vi "Localization Mockup.vi"() -> ()   [LabVIEW 2015, in "Localization Mockup.lvlib"]
uses:
  Localization Mockup.lvlib
  PathfindingSettings.ctl
  MovementSettings.ctl
  PathCostWeights.ctl
  IntermediatePositionGrids.ctl
  Move.ctl
  <vilib>/Utility/miscctls.llb/LVBoundsTypeDef.ctl
  <vilib>/Utility/inputDevices.llb/mouseAcquire.vi
  Navigation2017-SubVIs.lvlib
  Navigation2017-util.lvlib
  Navigation2017.lvlib
panel:
  out "Heartbeat":bool=TRUE
  out "Move":T1={"Did Reach Dest"=FALSE, "Did Collide"=FALSE, "Sum of Angle Changes (rad)"=0.0, "Move Length (m)"=0.0, "Closeness Sum"=0.0, "Positions Along Move"=[{"x"=0.9948666606172851, "y"=1.2473033614636722, "angle"=1.6518517499971999}, {"x"=1.001713061664076, "y"=1.44718614409566, "angle"=1.536557632350141}, {"x"=1.031508296522137, "y"=1.644954301238697, "angle"=1.4212635147030823}, {"x"=1.0838567436054756, "y"=1.8379818642652317, "angle"=1.3059693970560236}, {"x"=1.158063319429836, "y"=2.0237058102291905, "angle"=1.1906752794089648}, {"x"=1.2531427079418764, "y"=2.199660093724013, "angle"=1.075381161761906}, {"x"=1.3678324435608575, "y"=2.363508391071432, "angle"=0.9600870441148471}, {"x"=1.5006096742160095, "y"=2.5130751220631486, "angle"=0.8447929264677883}, {"x"=1.6497113817997135, "y"=2.6463743373482496, "angle"=0.7294988088207294}, {"x"=1.8131577915490082, "y"=2.7616360878991832, "angle"=0.6142046911736705}, {"x"=1.988778659525295, "y"=2.8573299264221292, "angle"=0.49891057352661167}, {"x"=2.1742420891466807, "y"=2.9321852286596677, "angle"=0.38361645587955284}, {"x"=2.367085494146603, "y"=2.9852080647591808, "angle"=0.268322338232494}, {"x"=2.564748296832094, "y"=3.0156943966887, "angle"=0.1530282205854352}, {"x"=2.7646059274737063, "y"=3.0232394264647042, "angle"=0.037734102938376354}, {"x"=2.9640046733826884, "y"=3.007742971065964, "angle"=-0.07756001470868248}, {"x"=3.1602969149488147, "y"=2.969410792665233, "angle"=-0.19285413235574134}, {"x"=3.350876280774229, "y"=2.90875186651596, "angle"=-0.30814825000280016}, {"x"=3.5332122551128893, "y"=2.8265716227710582, "angle"=-0.423442367649859}, {"x"=3.704883778097503, "y"=2.7239612519689644, "angle"=-0.5387364852969179}, {"x"=3.863611392609625, "y"=2.6022832161889142, "angle"=-0.6540306029439767}, {"x"=4.007287510946279, "y"=2.4631531582585313, "angle"=-0.7693247205910356}, {"x"=4.134004399401844, "y"=2.3084184492235513, "angle"=-0.8846188382380945}, {"x"=4.134004399401844, "y"=2.3084184492235513, "angle"=5.398566468941492}], "Moved Fwd"=TRUE}
  in  "Specify End Angle":bool
  in  "Pathfinding Settings":T2={"Movement Settings"={"Arrival Tolerance (m)"=0.01, "Closeness Threshold (m)"=0.5, "Pit Obstacle Radius (m)"=0.5, "Pit Locations"=[]}, "Dead Zone"=0.75, "Max Moves"=3.0, "Move Segment Length (m)"=0.2, "Path Cost Weights"={"Length Weight"=1.0, "Angle Weight"=0.0, "Angle Error Weight"=1000.0, "Angle Error Threshold"=0.314, "Per Move Penalty"=0.05, "Closeness Weight"=100.0, "Too Short Penalty"=100.0, "Too Short Threshold"=1.5}, "Desperation - Reduction Per Attempt (Ratio)"=0.9, "Desperation - Max Attempts"=1, "Log All Move Points"=FALSE, "Intermediate Position Grids"=[{"x1"=0.0, "x2"=1.75, "resolution"=0.15}, {"x1"=1.75, "x2"=7.38, "resolution"=0.4}]}
  in  "Full Pathfinding":bool=TRUE
  in  "Choose Background":u16
  out "Numeric 4":dbl=2.9395922017001697
  out "Numeric 3":dbl=2.276578752456705
  out "Numeric 2":dbl=2.7971305825546784
  out "Numeric":dbl=2.0893893844143916
  in  "Speed":dbl(slide) scale=0.0..1.0
  in  "Turning Radius":dbl(slide)=1.7346938775510203 scale=1.0..10.0
  out "Dest Y":dbl
  out "Dest X":dbl
  in  "ACTUALLY SEND VALUES TO ROBOT":bool
  in  "Send Robot STOP, end program":bool
  out "Left Side PWM":dbl=0.5
  out "Right Side PWM":dbl=0.5
  out "Bot Y (m)":dbl=1.04796
  out "Bot X (m)":dbl=1.01106
  out "Mouse Button Down":dbl
  out "Mouse Down":bool
  out "Bot Angle":dbl=1.7671458676442586
  out "Mouse Y (m)":dbl
  out "Mouse X (m)":dbl=0.08856
  out "Arena Control - DO NOT MOVE":picture
  # "\"missing\" side of robot faces forward (i.e. camera-side, boxes in back)"
  # "CONTROLS:\nClick + Drag to Move Robot\nMouse Wheel to Spin Robot\nRight Click to Place Yellow Destination Puck"
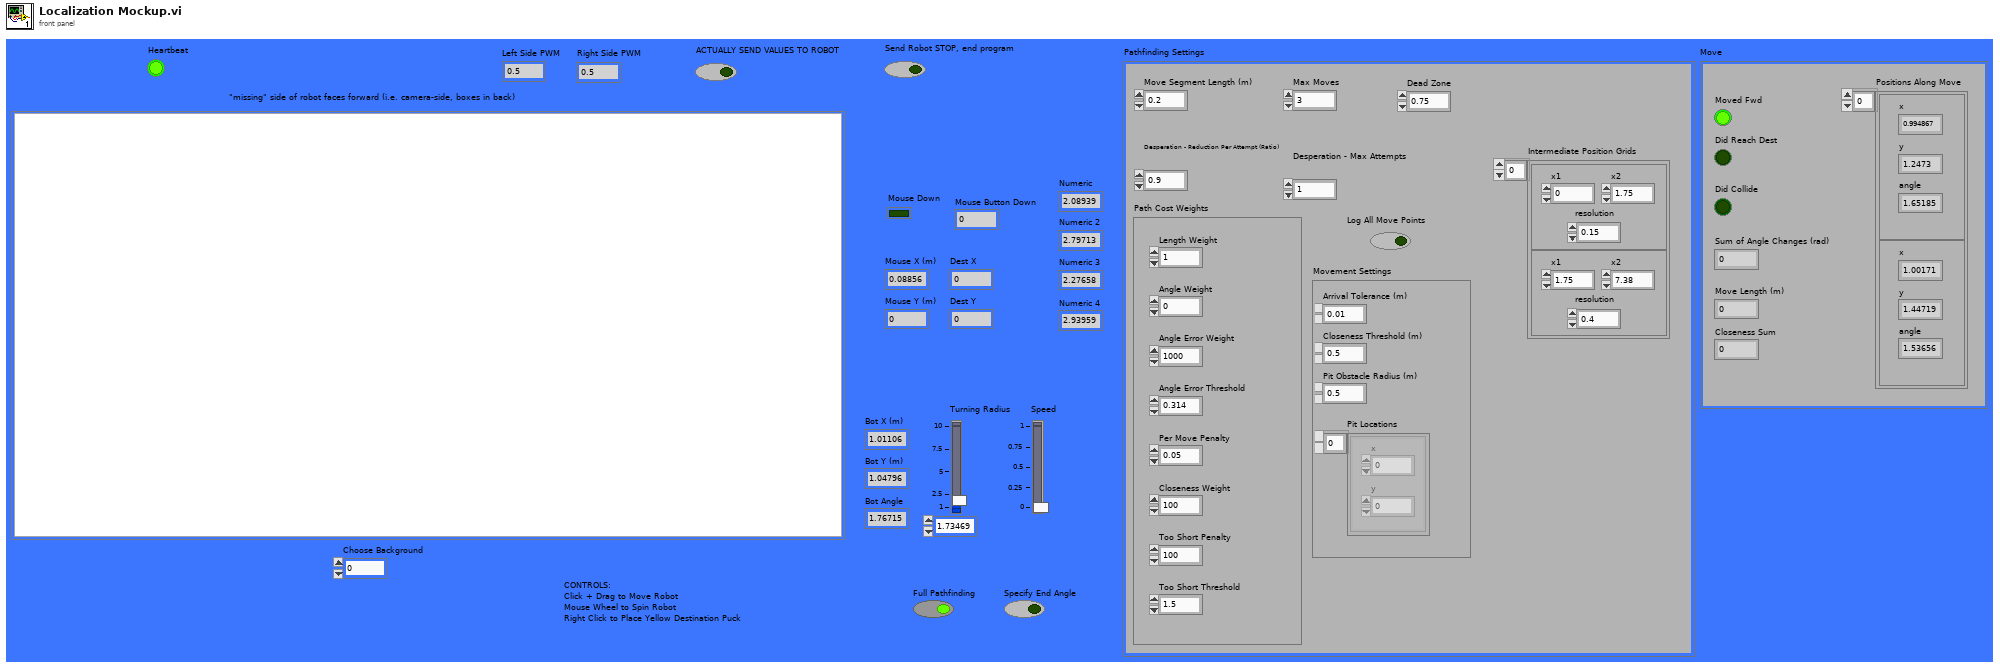
[diagram p1: front panel]
types:
  T1 = typedef "Navigation2017.lvlib/Move.ctl" = cluster{"Did Reach Dest":bool, "Did Collide":bool, "Sum of Angle Changes (rad)":dbl, "Move Length (m)":dbl, "Closeness Sum":dbl, "Positions Along Move":cluster{"x":dbl, "y":dbl, "angle":dbl}[], "Moved Fwd":bool}
  T2 = typedef "Navigation2017.lvlib/PathfindingSettings.ctl" = cluster{"Movement Settings":T3, "Dead Zone":dbl, "Max Moves":dbl, "Move Segment Length (m)":dbl, "Path Cost Weights":T4, "Desperation - Reduction Per Attempt (Ratio)":dbl, "Desperation - Max Attempts":i16, "Log All Move Points":bool, "Intermediate Position Grids":T5}
  T3 = typedef "Navigation2017.lvlib/MovementSettings.ctl" = cluster{"Arrival Tolerance (m)":dbl, "Closeness Threshold (m)":dbl, "Pit Obstacle Radius (m)":dbl, "Pit Locations":cluster{"x":dbl, "y":dbl}[]}
  T4 = typedef "Navigation2017.lvlib/PathCostWeights.ctl" = cluster{"Length Weight":dbl, "Angle Weight":dbl, "Angle Error Weight":dbl, "Angle Error Threshold":dbl, "Per Move Penalty":dbl, "Closeness Weight":dbl, "Too Short Penalty":dbl, "Too Short Threshold":dbl}
  T5 = typedef "Navigation2017.lvlib/IntermediatePositionGrids.ctl" = cluster{"x1":dbl, "x2":dbl, "resolution":dbl}[]
  T6 = typedef "LVBoundsTypeDef.ctl" = cluster{"Width":u32, "Height":u32}
  T7 = typedef "imagedata.ctl" = cluster{"image type":i32, "image depth":i32, "image":u8[], "mask":u8[], "colors":u32[], "Rectangle":cluster{"left":i16, "top":i16, "right":i16, "bottom":i16}}
  T8 = cluster{"Width":u16, "Style":enum32{"Solid", "Dash", "Dot", "DashDot", "DashDotDot"}}
  T9 = cluster{"Arrival Tolerance (m)":dbl, "Closeness Threshold (m)":dbl, "Pit Obstacle Radius (m)":dbl, "Pit Locations":cluster{"x":dbl, "y":dbl}[]}
  T10 = cluster{"Horizontal":i32, "Vertical":i32, "Scrolling":i32}
  T11 = typedef "LVRectTypeDef.ctl" = cluster{"Left":i16, "Top":i16, "Right":i16, "Bottom":i16}
  T12 = typedef "LVPointTypeDef.ctl" = cluster{"Horizontal":i16, "Vertical":i16}
  T13 = typedef "LVPositionTypeDef.ctl" = cluster{"Left":i32, "Top":i32}
  T14 = cluster{"Mouse X (m)":dbl, "Mouse Y (m)":dbl, dbl}
  T15 = typedef "Navigation2017.lvlib/Path.ctl" = cluster{"Dest Angle Error":dbl, "Dest Angle Considered":bool, "Moves":T1[]}
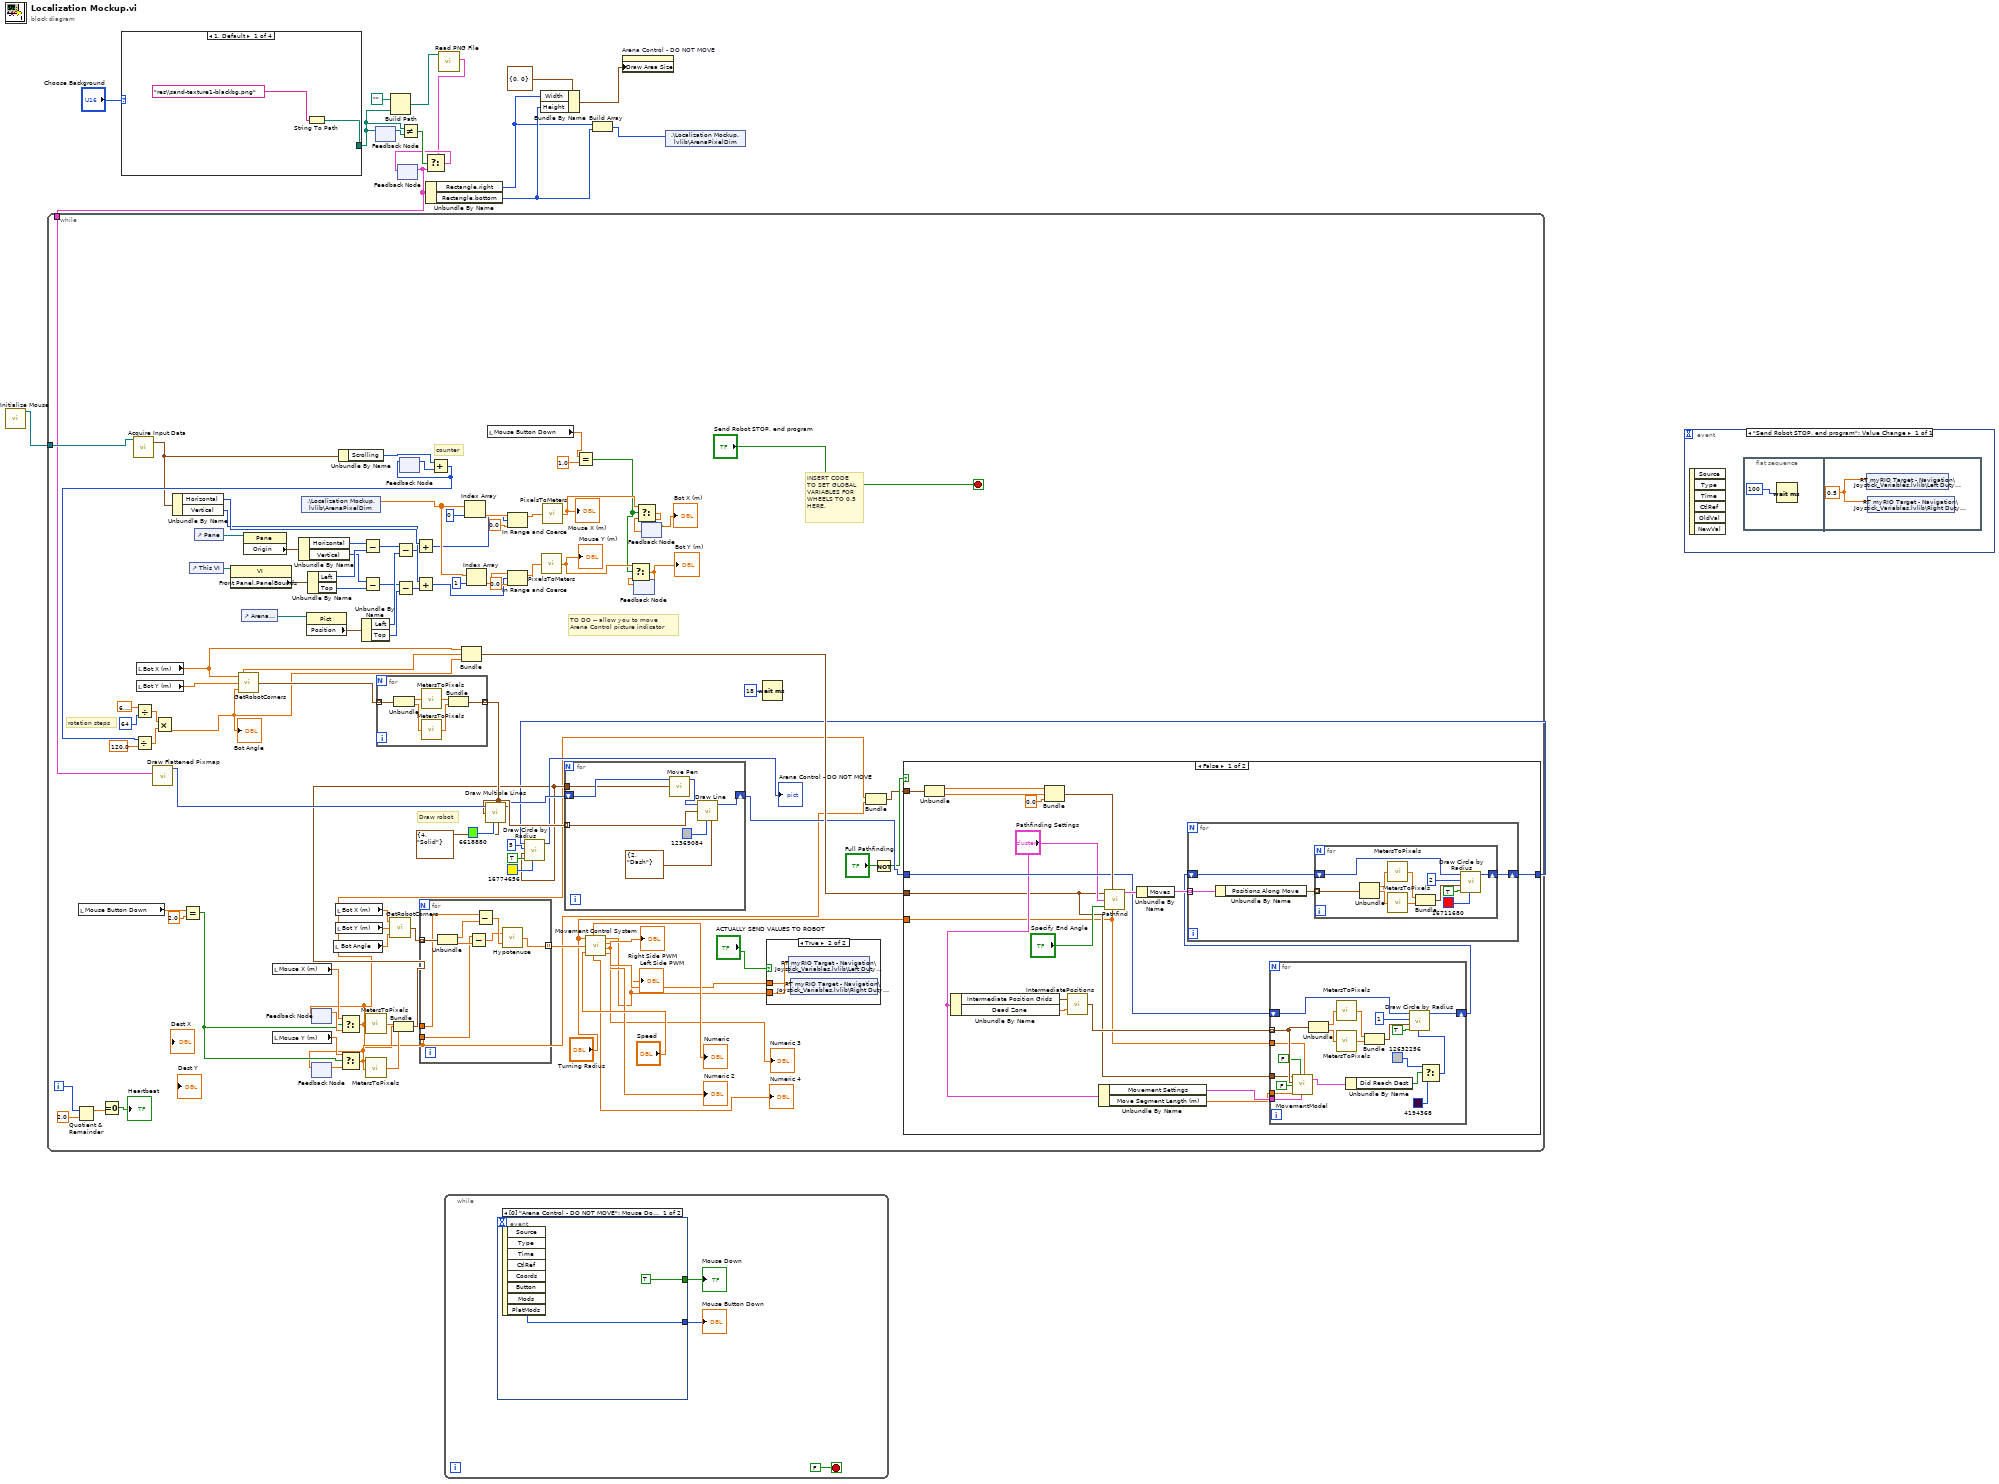
[diagram p0: block diagram]
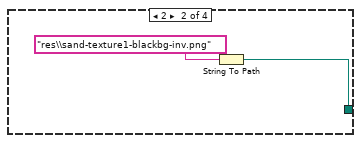
[diagram p2: hidden frame]
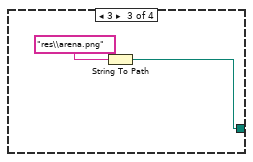
[diagram p3: hidden frame]
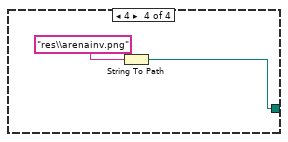
[diagram p4: hidden frame]
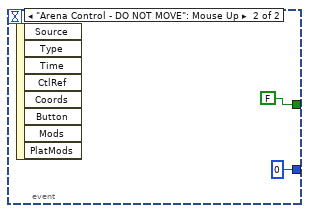
[diagram p5: hidden frame]
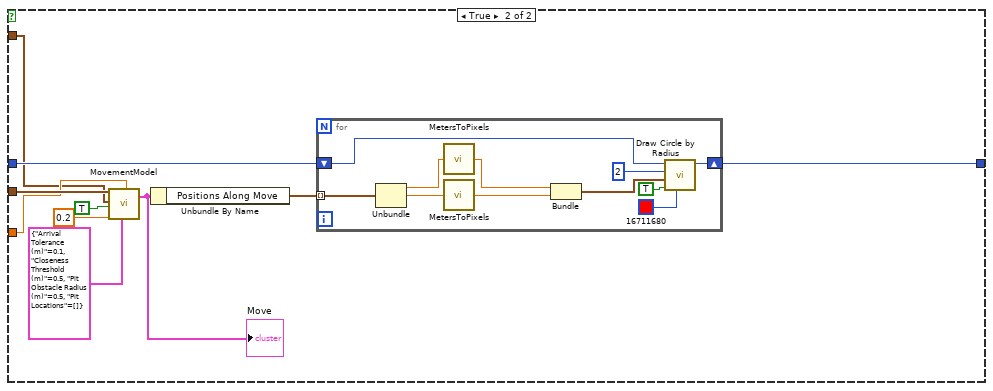
[diagram p6: hidden frame]
diagram:
  n1 = call <vilib>:"Initialize Mouse.vi"() -> ("device ID"=w15:refnum<k1>)  [unwired: 10 in, 1 out]
  n2 = case shown="1, Default" "Choose Background" {
    tunnel: [w16 w18 w20 w22] -> w10
    frame 1, Default {
      n3 = String To Path(string="res\\sand-texture1-blackbg.png" ("name or relative path")) -> (path=w16:path)
    }
    frame 2 {
      n4 = String To Path(string="res\\sand-texture1-blackbg-inv.png" ("name or relative path")) -> (path=w18:path)
    }
    frame 3 {
      n5 = String To Path(string="res\\arena.png" ("name or relative path")) -> (path=w20:path)
    }
    frame 4 {
      n6 = String To Path(string="res\\arenainv.png" ("name or relative path")) -> (path=w22:path)
    }
  }
  n7 = feedback #1() -> (w11:path)  [unwired: 1 in]
  n8 = feedback-in #1(w10) -> ()
  n9 = Build Path(base path=path "", name or relative path=w10) -> (appended path=w2:path)
  n10 = feedback #2() -> (w1:T7)  [unwired: 1 in]
  n11 = while {
    tunnel: w15 -> [w123]
    tunnel: w1 -> [w42]
    i -> [w34]
    stop <- "Send Robot STOP, end program" stop-if-true
    # "TO DO -- allow you to move\nArena Control picture indicator"
    # "INSERT CODE\nTO SET GLOBAL\nVARIABLES FOR\nWHEELS TO 0.5\nHERE."
    # "Draw robot"
    # "rotation steps"
    # "counter"
    n12 = Quotient & Remainder(x=w34, y=2.0) -> (x-y*floor(x/y)=w33:dbl)  [unwired: 1 out]
    n13 = local read "Mouse Button Down"() -> (w81:dbl)
    n14 = Equal To 0?(x=w33) -> (x = 0?=→"Heartbeat":bool)
    n15 = call-poly <vilib>:"Acquire Input Data.vi"("device ID"=w123) -> ("axis info"=w25:T10)  [unwired: 15 in, 3 out]
    n16 = Divide(x=6.283185307179586, y=64) -> (x/y=w95:dbl)
    n17 = local read "Bot X (m)"() -> (w49:dbl)
    n18 = local read "Bot Y (m)"() -> (w48:dbl)
    n19 = call <vilib>:"Draw Flattened Pixmap.vi"("image data"=w42) -> ("new picture"=w104:picture)  [unwired: 8 in]
    n20 = Unbundle By Name(w25) -> ("Horizontal"=w114:i32, "Vertical"=w113:i32)
    n21 = Equal?(x=w81, y=2.0) -> (x = y?=w71:bool)
    n22 = control-ref of="This VI"() -> (w61:refnum<vi>)
    n23 = control-ref of="Pane"() -> (w121:refnum<vi>)
    n24 = property class="VI"(reference=w61) -> ("Front Panel.PanelBounds"=w119:T11)  [unwired: 1 in, 2 out]
    n25 = control-ref of="Arena Control"() -> (w60:refnum<vi>)
    n26 = property class="Pane"(reference=w121) -> ("Origin"=w120:T12)  [unwired: 1 in, 2 out]
    n27 = local read "Mouse X (m)"() -> (w72:dbl)
    n28 = local read "Mouse Y (m)"() -> (w73:dbl)
    n29 = Unbundle By Name(w120) -> ("Horizontal"=w118:i16, "Vertical"=w116:i16)
    n30 = shared-variable ".\\Localization Mockup.lvlib\\ArenaPixelDim"() -> (w108:dbl[])  [unwired: 1 in, 1 out]
    n31 = property class="Pict"(reference=w60) -> ("Position"=w59:T13)  [unwired: 1 in, 2 out]
    n32 = Unbundle By Name(w119) -> ("Left"=w117:i16, "Top"=w115:i16)
    n33 = feedback #3() -> (w80:dbl)  [unwired: 1 in]
    n34 = feedback #4() -> (w79:dbl)  [unwired: 1 in]
    n35 = local read "Bot Angle"() -> (w76:dbl)
    n36 = local read "Bot X (m)"() -> (w69:dbl)
    n37 = local read "Bot Y (m)"() -> (w70:dbl)
    n38 = Unbundle By Name(w25) -> ("Scrolling"=w24:i32)
    n39 = Select(t=w72, s=w71, f=w80) -> (s? t:f=w37:dbl)
    n40 = feedback-in #3(w37) -> ()
    n41 = Select(t=w73, s=w71, f=w79) -> (s? t:f=w38:dbl)
    n42 = feedback-in #4(w38) -> ()
    n43 = Unbundle By Name(w59) -> ("Left"=w29:i32, "Top"=w26:i32)
    n44 = Subtract(x=w118, y=w117) -> (x-y=w30:i16)
    n45 = Subtract(x=w116, y=w115) -> (x-y=w27:i16)
    n46 = call "MetersToPixels.vi"("Arena Meters"=w37) -> ("Arena Pixels"=w64:dbl)
    n47 = call "MetersToPixels.vi"("Arena Meters"=w38) -> ("Arena Pixels"=w65:dbl)
    n48 = call "GetRobotCorners.vi"("botAngle (rad)"=w76, "botY (m)"=w70, "botX (m)"=w69) -> ("Corner Points (m)"=w78:cluster{dbl, dbl}[])
    n49 = Bundle("Arena Pixels"=w64, "Arena Pixels"=w65) -> (w45:cluster{"Arena Pixels":dbl, "Arena Pixels":dbl})  [unwired: 1 in]
    n50 = Subtract(x=w30, y=w29) -> (x-y=w31:i32)
    n51 = Subtract(x=w27, y=w26) -> (x-y=w28:i32)
    n52 = feedback #5() -> (w122:i32)  [unwired: 1 in]
    n53 = Add(x=w114, y=w31) -> (x+y=w58:i32)
    n54 = Add(x=w113, y=w28) -> (x+y=w57:i32)
    n55 = for {
      tunnel: w78 -> [w209] mode=indexing
      tunnel: [w204] -> w77 mode=indexing
      tunnel: w37 -> [w203]
      tunnel: w38 -> [w202]
      n56 = Unbundle(w209) -> (w208:dbl, w205:dbl)
      n57 = Subtract(x=w202, y=w205) -> (x-y=w206:dbl)
      n58 = Subtract(x=w203, y=w208) -> (x-y=w207:dbl)
      n59 = call "Hypotenuse.vi"("y"=w207, "x"=w206) -> ("r"=w204:dbl)
    }
    n60 = Add(x=w24, y=w122) -> (x+y=w94:i32)
    n61 = Divide(x=w94, y=120.0) -> (x/y=w101:dbl)
    n62 = Multiply(x=w95, y=w101) -> (x*y=w47:dbl)
    "Bot Angle" <- w47
    n63 = call "GetRobotCorners.vi"("botAngle (rad)"=w47, "botY (m)"=w48, "botX (m)"=w49) -> ("Corner Points (m)"=w93:cluster{dbl, dbl}[])
    n64 = for {
      tunnel: [w222] -> w92 mode=indexing
      tunnel: w93 -> [w221] mode=indexing
      n65 = Unbundle(w221) -> (w220:dbl, w217:dbl)
      n66 = call "MetersToPixels.vi"("Arena Meters"=w220) -> ("Arena Pixels"=w219:dbl)
      n67 = call "MetersToPixels.vi"("Arena Meters"=w217) -> ("Arena Pixels"=w218:dbl)
      n68 = Bundle("Arena Pixels"=w219, "Arena Pixels"=w218) -> (w222:cluster{"Arena Pixels":dbl, "Arena Pixels":dbl})  [unwired: 1 in]
    }
    n69 = feedback-in #5(w94) -> ()
    n70 = Bundle("Bot X (m)"=w49, "Bot Y (m)"=w48, w47) -> (w46:cluster{"Bot X (m)":dbl, "Bot Y (m)":dbl, dbl})  [unwired: 1 in]
    n71 = Index Array(array=w108, index=0) -> (element=w110:dbl)
    n72 = Index Array(array=w108, index=1) -> (element=w106:dbl)
    n73 = call <vilib>:"Draw Multiple Lines.vi"("picture"=w104, "line endpoints"=w92, "color(black)"=u32 6618880, "pen"=T8 {"Width"=4, "Style"=enum."Solid"}) -> ("new picture"=w63:picture)  [unwired: 5 in]
    n74 = local read "Mouse Button Down"() -> (w90:dbl)
    n75 = In Range and Coerce(upper limit=w110, x=w58, lower limit=0.0) -> (coerced(x)=w100:dbl)  [unwired: 1 out]
    n76 = In Range and Coerce(upper limit=w106, x=w57, lower limit=0.0) -> (coerced(x)=w99:dbl)  [unwired: 1 out]
    n77 = call "PixelsToMeters.vi"("Arena Meters"=w99) -> ("Arena Pixels"=w85:dbl)
    "Mouse Y (m)" <- w85
    n78 = call "PixelsToMeters.vi"("Arena Meters"=w100) -> ("Arena Pixels"=w89:dbl)
    "Mouse X (m)" <- w89
    n79 = for {
      tunnel: w92 -> [w213] mode=indexing
      shift-right: [w214] -> w43
      shift-left: w63 -> [w215]
      tunnel: w45 -> [w210]
      n80 = call <vilib>:"Move Pen.vi"("new position"=w210, "picture"=w215) -> ("new picture"=w216:picture)  [unwired: 3 in]
      n81 = call <vilib>:"Draw Line.vi"("picture"=w216, "end point"=w213, "color(black)"=u32 12369084, "pen"=T8 {"Width"=2, "Style"=enum."Dash"}) -> ("new picture"=w214:picture)  [unwired: 5 in]
    }
    n82 = Equal?(x=w90, y=1.0) -> (x = y?=w84:bool)
    n83 = call "Movement Control System.vi"("Turning Radius"="Turning Radius", "Corner Distances"=w77, "Speed"="Speed") -> ("Corner Dist 1"=→"Numeric":dbl, "Corner Dist 4"=→"Numeric 4":dbl, "Left Side PWM"=w51:dbl, "Corner Dist 2"=→"Numeric 2":dbl, "Right Side PWM"=w54:dbl, "Corner Dist 3"=→"Numeric 3":dbl)
    "Right Side PWM" <- w54
    "Left Side PWM" <- w51
    n84 = feedback #6() -> (w88:dbl)  [unwired: 1 in]
    n85 = Select(t=w85, s=w84, f=w88) -> (s? t:f=w83:dbl)
    "Bot Y (m)" <- w83
    n86 = feedback-in #6(w83) -> ()
    n87 = feedback #7() -> (w86:dbl)  [unwired: 1 in]
    "Bot X (m)" <- w86
    n88 = Select(t=w89, s=w84, f=w86) -> (s? t:f=w87:dbl)
    n89 = feedback-in #7(w87) -> ()
    n90 = Wait (ms)(milliseconds to wait=u32 18) -> ()  [unwired: 1 out]
    n91 = case shown="True" "ACTUALLY SEND VALUES TO ROBOT" {
      tunnel: w51 -> [_ w201]
      tunnel: w54 -> [_ w200]
      frame False {
      }
      frame True {
        n92 = shared-variable "RT myRIO Target - Navigation\\Joystick_Variables.lvlib\\Left Duty Cycle"(w201) -> ()  [unwired: 1 in, 1 out]
        n93 = shared-variable "RT myRIO Target - Navigation\\Joystick_Variables.lvlib\\Right Duty Cycle"(w200) -> ()  [unwired: 1 in, 1 out]
      }
    }
    n94 = Bundle("Mouse X (m)"=w37, "Mouse Y (m)"=w38) -> (w36:cluster{"Mouse X (m)":dbl, "Mouse Y (m)":dbl})  [unwired: 1 in]
    n95 = Not(x="Full Pathfinding") -> (.not. x?=w39:bool)
    n96 = case shown="False" w39 {
      tunnel: w46 -> [w125 w188]
      tunnel: [w142 w187] -> w44
      tunnel: w43 -> [w132 w186]
      tunnel: "Turning Radius" -> [w124 w181]
      tunnel: w36 -> [w136 w180]
      frame False {
        n97 = Unbundle(w136) -> ("Mouse X (m)"=w137:dbl, "Mouse Y (m)"=w135:dbl)
        n98 = Unbundle By Name("Pathfinding Settings") -> ("Intermediate Position Grids"=w130:T5, "Dead Zone"=w129:dbl)
        n99 = Bundle("Mouse X (m)"=w137, "Mouse Y (m)"=w135, 0.0) -> (w138:T14)  [unwired: 1 in]
        n100 = call "IntermediatePositions.vi"("Dead Zone"=w129, "Position Grids"=w130) -> ("Positions"=w131:cluster{dbl, dbl}[])
        n101 = Unbundle By Name("Pathfinding Settings") -> ("Movement Settings"=w127:T3, "Move Segment Length (m)"=w126:dbl)
        n102 = call "Pathfind.vi"("Start Vector"=w125, "Destination"=w138, "Pathfinding Settings"="Pathfinding Settings", "Specified End Angle"="Specify End Angle", "Turn Radius (m)"=w124) -> ("Best Path"=w141:T15)  [unwired: 3 out]
        n103 = Unbundle By Name(w141) -> ("Moves"=w140:T1[])
        n104 = for {
          shift-right: [w163] -> w133
          shift-left: w132 -> [w162]
          tunnel: w131 -> [w146] mode=indexing
          tunnel: w127 -> [w149]
          tunnel: w126 -> [w148]
          tunnel: w125 -> [w145]
          tunnel: w124 -> [w143]
          n105 = call "MovementModel.vi"("Start Vector"=w145, "Destination"=w146, "Log All Points"=FALSE, "Segment Length (m)"=w148, "Do Force Direction"=FALSE, "Movement Settings"=w149, "Turn Radius (m)"=w143) -> ("Move"=w154:T1)  [unwired: 11 in, 1 out]
          n106 = Unbundle(w146) -> (w159:dbl, w158:dbl)
          n107 = call "MetersToPixels.vi"("Arena Meters"=w159) -> ("Arena Pixels"=w157:dbl)
          n108 = call "MetersToPixels.vi"("Arena Meters"=w158) -> ("Arena Pixels"=w156:dbl)
          n109 = Unbundle By Name(w154) -> ("Did Reach Dest"=w153:bool)
          n110 = Bundle("Arena Pixels"=w157, "Arena Pixels"=w156) -> (w155:cluster{"Arena Pixels":dbl, "Arena Pixels":dbl})  [unwired: 1 in]
          n111 = Select(t=u32 12632256 ("color(black)"), s=w153, f=u32 4194368 ("color(black)")) -> (s? t:f=w151:u32)
          n112 = call <vilib>:"Draw Circle by Radius.vi"("color(black)"=w151, "fill?(F)"=TRUE, "pixel center"=w155, "radius"=i16 1, "picture"=w162) -> ("new picture"=w163:picture)  [unwired: 6 in]
        }
        n113 = for {
          shift-right: [w167] -> w142
          shift-left: w133 -> [w166]
          tunnel: w140 -> [w165] mode=indexing
          n114 = Unbundle By Name(w165) -> ("Positions Along Move"=w164:cluster{"x":dbl, "y":dbl, "angle":dbl}[])
          n115 = for {
            shift-right: [w175] -> w167
            shift-left: w166 -> [w174]
            tunnel: w164 -> [w173] mode=indexing
            n116 = Unbundle(w173) -> ("x"=w172:dbl, "y"=w171:dbl)  [unwired: 1 out]
            n117 = call "MetersToPixels.vi"("Arena Meters"=w172) -> ("Arena Pixels"=w170:dbl)
            n118 = call "MetersToPixels.vi"("Arena Meters"=w171) -> ("Arena Pixels"=w169:dbl)
            n119 = Bundle("Arena Pixels"=w170, "Arena Pixels"=w169) -> (w168:cluster{"Arena Pixels":dbl, "Arena Pixels":dbl})  [unwired: 1 in]
            n120 = call <vilib>:"Draw Circle by Radius.vi"("color(black)"=u32 16711680, "fill?(F)"=TRUE, "pixel center"=w168, "radius"=i16 2, "picture"=w174) -> ("new picture"=w175:picture)  [unwired: 6 in]
          }
        }
      }
      frame True {
        n121 = call "MovementModel.vi"("Start Vector"=w188, "Destination"=w180, "Log All Points"=TRUE, "Segment Length (m)"=0.2, "Movement Settings"=T9 {"Arrival Tolerance (m)"=0.1, "Closeness Threshold (m)"=0.5, "Pit Obstacle Radius (m)"=0.5, "Pit Locations"=[]}, "Turn Radius (m)"=w181) -> ("Move"=w184:T1)  [unwired: 12 in, 1 out]
        "Move" <- w184
        n122 = Unbundle By Name(w184) -> ("Positions Along Move"=w185:cluster{"x":dbl, "y":dbl, "angle":dbl}[])
        n123 = for {
          shift-right: [w196] -> w187
          shift-left: w186 -> [w195]
          tunnel: w185 -> [w194] mode=indexing
          n124 = Unbundle(w194) -> ("x"=w193:dbl, "y"=w192:dbl)  [unwired: 1 out]
          n125 = call "MetersToPixels.vi"("Arena Meters"=w193) -> ("Arena Pixels"=w191:dbl)
          n126 = call "MetersToPixels.vi"("Arena Meters"=w192) -> ("Arena Pixels"=w190:dbl)
          n127 = Bundle("Arena Pixels"=w191, "Arena Pixels"=w190) -> (w189:cluster{"Arena Pixels":dbl, "Arena Pixels":dbl})  [unwired: 1 in]
          n128 = call <vilib>:"Draw Circle by Radius.vi"("color(black)"=u32 16711680, "fill?(F)"=TRUE, "pixel center"=w189, "radius"=i16 2, "picture"=w195) -> ("new picture"=w196:picture)  [unwired: 6 in]
        }
      }
    }
    n129 = call <vilib>:"Draw Circle by Radius.vi"("color(black)"=u32 16774656, "fill?(F)"=TRUE, "pixel center"=w45, "radius"=i16 5, "picture"=w44) -> ("new picture"=→"Arena Control - DO NOT MOVE":picture)  [unwired: 6 in]
  }
  n130 = Not Equal?(x=w10, y=w11) -> (x != y?=w14:bool)
  n131 = Unbundle By Name(w1) -> ("Rectangle.right"=w6:i16, "Rectangle.bottom"=w7:i16)
  n132 = call <vilib>:"Read PNG File.vi"("path to PNG file"=w2) -> ("image data"=w12:T7)  [unwired: 8 in, 2 out]
  n133 = Select(t=w12, s=w14, f=w1) -> (s? t:f=w13:T7)
  n134 = feedback-in #2(w13) -> ()
  n135 = while {
    stop <- FALSE stop-if-true
    n136 = event shown="[0] \"Arena Control - DO NOT MOVE\": Mouse Down" {
      selector: _ -> [_ _]
      dyn-events: _ -> [_ _]
      timeout: _ -> [_ _]
      tunnel: [w226 u16 0 ("Button")] -> w225
      tunnel: [TRUE FALSE] -> w224
      event "Arena Control - DO NOT MOVE": Mouse Down {
        n137 = event-data() -> ("Button"=w226:u16)  [unwired: 1 in, 7 out]
      }
      event "Arena Control - DO NOT MOVE": Mouse Up {
        n138 = event-data() -> ()  [unwired: 1 in, 8 out]
      }
    }
    "Mouse Down" <- w224
    "Mouse Button Down" <- w225
  }
  n139 = Bundle By Name(cluster=T6 {"Width"=0, "Height"=0} ("Draw Area Size"), "Width"=w6, "Height"=w7) -> (w8:T6)
  n140 = Build Array(w6, w7) -> (w5:i16[])
  n141 = property on="Arena Control - DO NOT MOVE" class="Pict"("Draw Area Size"=w8) -> ()  [unwired: 2 in, 2 out]
  n142 = shared-variable ".\\Localization Mockup.lvlib\\ArenaPixelDim"(w5) -> ()  [unwired: 1 in, 1 out]
  n143 = event shown="[0] \"Send Robot STOP, end program\": Value Change" {
    selector: _ -> [_]
    dyn-events: _ -> [_]
    timeout: _ -> [_]
    event "Send Robot STOP, end program": Value Change {
      n144 = event-data() -> ()  [unwired: 1 in, 6 out]
      n145 = flat-sequence {
        frame #0 {
          n146 = Wait (ms)(milliseconds to wait=u32 100) -> ()  [unwired: 1 out]
        }
        frame #1 {
          w231 = 0.5
          n147 = shared-variable "RT myRIO Target - Navigation\\Joystick_Variables.lvlib\\Left Duty Cycle"(w231) -> ()  [unwired: 1 in, 1 out]
          n148 = shared-variable "RT myRIO Target - Navigation\\Joystick_Variables.lvlib\\Right Duty Cycle"(w231) -> ()  [unwired: 1 in, 1 out]
        }
      }
    }
  }
